vi "Read Position.vi"(8 "error in (no error)":errorcluster, 11 "I2C Accelerometer Gyro in":refnum<class "I2C Accelerometer Gyro.lvclass">) -> (0 "error out":errorcluster, 2 "Position":dbl[](array[numeric]) format="%.2f", 3 "I2C Accelerometer Gyro out":refnum<class "I2C Accelerometer Gyro.lvclass">)   [LabVIEW 2020, in "CTI-Peripheral.lvlib" / "I2C Accelerometer Gyro.lvclass"]
uses:
  I2C Accelerometer Gyro.lvclass
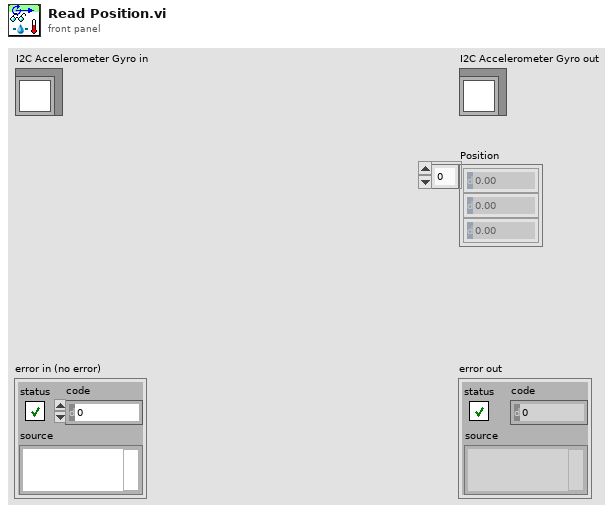
[diagram p1: front panel]
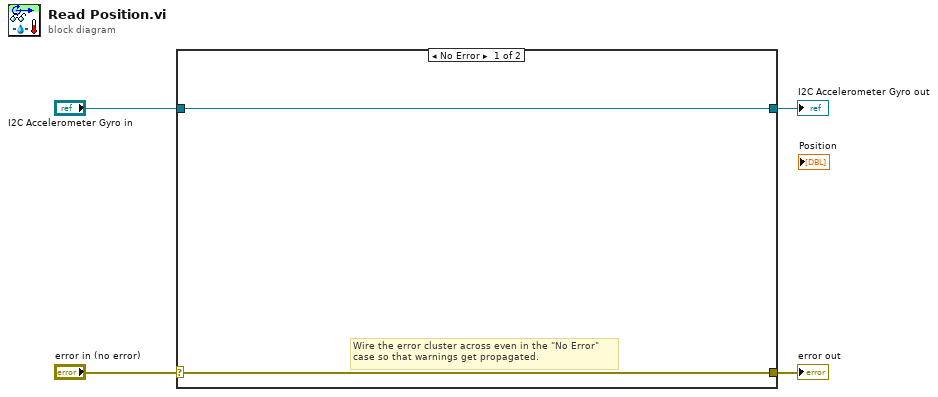
[diagram p0: block diagram]
diagram:
  n1 = case shown="No Error" "error in (no error)" {
    selector: "error in (no error)" -> [w5 w8]
    tunnel: [w5 w8] -> w3
    tunnel: [w6 w7] -> w1
    tunnel: "I2C Accelerometer Gyro in" -> [w6 w7]
    frame No Error {
      # "Wire the error cluster across even in the \"No Error\"\ncase so that warnings get propagated."
    }
    frame Error {
    }
  }
  "error out" <- w3
  "I2C Accelerometer Gyro out" <- w1
